vi "SDSU_DACS_ReadConstants.vi"(8 "error in (no error)":errorcluster, 11 "file path":path=path "/home/arcconfig/DHE_DACS.cfg") -> (0 "error out":errorcluster, 1 "number of dacs":i32, 2 "constants":string[][](table), 3 "resolutions":string[][](table), 4 "resolution":i32=4095)   [LabVIEW 2016]
uses:
  <vilib>/Utility/config.llb/Read Key (String).vi
  <vilib>/Utility/config.llb/Read Key (I32).vi
  <vilib>/Utility/config.llb/NI_LVConfig.lvlib
panel:
  # "off"
  # "curr"
  # "ll"
  # "type"
  # "def"
  # "ul"
  # "ll"
  # "b"
  # "comment"
  # "dn"
  # "gain"
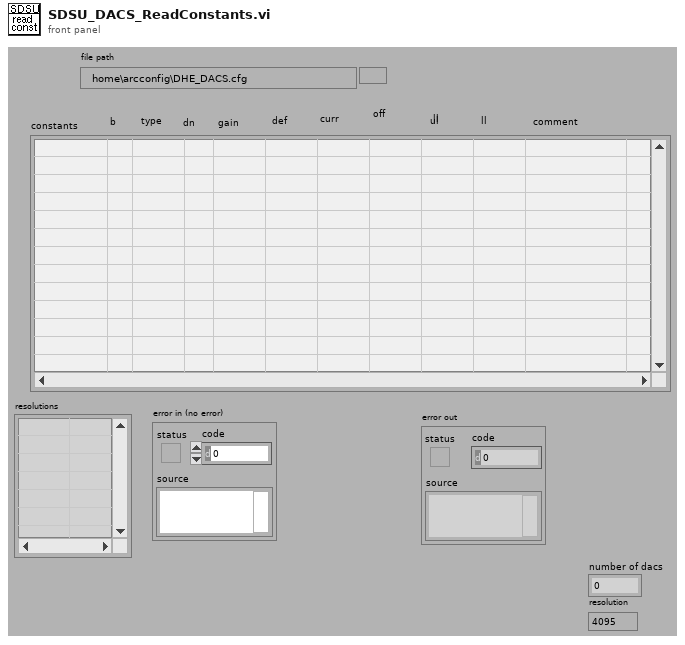
[diagram p1: front panel]
types:
  T1 = typedef "NI_LVConfig.lvlib/Config Data RefNum.ctl" = refnum<k1>
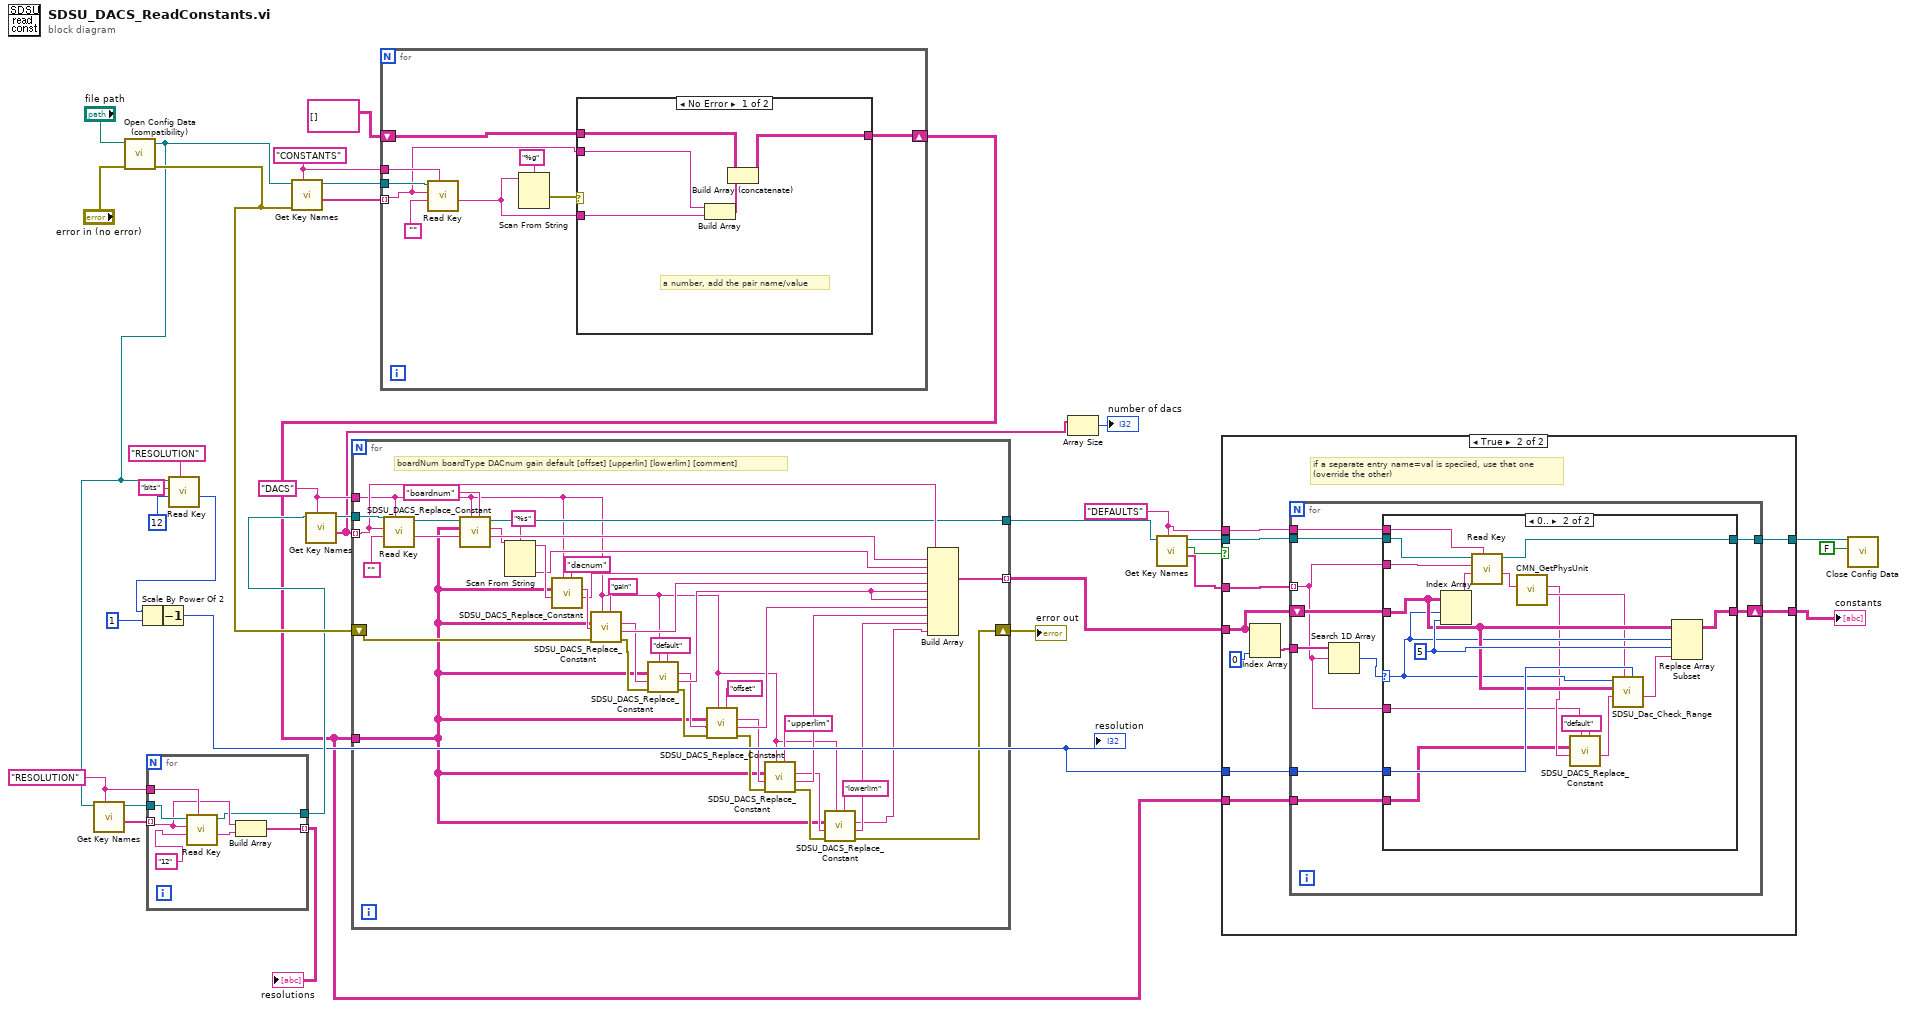
[diagram p0: block diagram]
diagram:
  w4 = "DEFAULTS" ("section")
  w14 = "RESOLUTION" ("section")
  w28 = "DACS" ("section")
  w35 = "CONSTANTS" ("section")
  n1 = call <vilib>:"Open Config Data (compatibility).vi"("error in (no error)"="error in (no error)", "configuration file path"="file path") -> ("error out"=w27:errorcluster, "refnum"=w16:T1)  [unwired: 7 in, 1 out]
  n2 = call <vilib>:"Get Key Names.vi"("section"=w14, "refnum"=w16) -> ("key names"=w15:string[], "refnum out"=w13:T1)  [unwired: 1 in, 7 out]
  n3 = for {
    tunnel: w15 -> [w38] mode=indexing
    tunnel: w14 -> [w42]
    tunnel: w13 -> [w40]
    tunnel: [w37] -> w11 mode=indexing
    tunnel: [w36] -> w12
    n4 = call-poly <vilib>:"Read Key.vi"("section"=w42, "default value"="12", "key"=w38, "refnum"=w40) -> ("value"=w39:string, "refnum out"=w36:T1)  [unwired: 2 in, 4 out]
    n5 = Build Array(w38, w39) -> (w37:string[])
  }
  "resolutions" <- w11
  n6 = call-poly <vilib>:"Read Key.vi"("section"="RESOLUTION", "default value"=12, "key"="bits", "refnum"=w16) -> ("value"=w20:i32)  [unwired: 1 in, 6 out]
  n7 = Scale By Power Of 2(n=w20, x=1) -> (x*2^n=w19:i32)
  n8 = Decrement(x=w19) -> (x-1=w2:i32)
  "resolution" <- w2
  n9 = call <vilib>:"Get Key Names.vi"("section"=w35, "error in (no error)"=w27, "refnum"=w16) -> ("key names"=w34:string[], "refnum out"=w31:T1)  [unwired: 7 out]
  n10 = call <vilib>:"Get Key Names.vi"("section"=w28, "refnum"=w12) -> ("key names"=w25:string[], "refnum out"=w29:T1)  [unwired: 1 in, 7 out]
  n11 = for {
    tunnel: w31 -> [w51]
    tunnel: w35 -> [w50]
    tunnel: w34 -> [w43] mode=indexing
    shift-right: [w48] -> w1
    shift-left: string[][] [] -> [w47]
    n12 = call-poly <vilib>:"Read Key.vi"("section"=w50, "default value"="", "key"=w43, "refnum"=w51) -> ("value"=w46:string)  [unwired: 2 in, 5 out]
    n13 = Scan From String(format string="%g", input string=w46) -> (error out=w44:errorcluster)  [unwired: 2 in, 4 out]
    n14 = case shown="No Error" w44 {
      tunnel: w43 -> [w56 _]
      tunnel: w46 -> [w55 _]
      tunnel: [w53 w57] -> w48
      tunnel: w47 -> [w52 w57]
      frame No Error {
        # "a number, add the pair name/value"
        n15 = Build Array(w56, w55) -> (w54:string[])
        n16 = Build Array (concatenate)(w52, w54) -> (w53:string[][])
      }
      frame Error {
        # "not a number\nskip it"
      }
    }
  }
  n17 = for {
    tunnel: w25 -> [w93] mode=indexing
    tunnel: w29 -> [w95]
    tunnel: w28 -> [w60]
    tunnel: [w88] -> w5 mode=indexing
    tunnel: w1 -> [w61]
    shift-right: [w75] -> w26
    shift-left: w27 -> [w91]
    tunnel: [w62] -> w10
    # "boardNum boardType DACnum gain default [offset] [upperlin] [lowerlim] [comment]"
    n18 = call-poly <vilib>:"Read Key.vi"("section"=w60, "default value"="", "key"=w93, "refnum"=w95) -> ("value"=w74:string, "refnum out"=w62:T1)  [unwired: 2 in, 4 out]
    n19 = call "SDSU_DACS_Replace_Constant.vi"("Field in"="boardnum", "DAC name"=w60, "value  in"=w74, "constants from file"=w61) -> ("value out"=w72:string, "rest out"=w71:string)  [unwired: 1 in, 5 out]
    n20 = Scan From String(format string="%s", input string=w71) -> (remaining string=w69:string, output 1=w68:string)  [unwired: 2 in, 3 out]
    n21 = call "SDSU_DACS_Replace_Constant.vi"("Field in"="dacnum", "DAC name"=w60, "value  in"=w69, "constants from file"=w61) -> ("value out"=w65:string, "rest out"=w66:string)  [unwired: 2 in, 4 out]
    n22 = call "SDSU_DACS_Replace_Constant.vi"("Field in"="gain", "DAC name"=w60, "error in (no error)"=w91, "value  in"=w66, "constants from file"=w61) -> ("error out"=w92:errorcluster, "value out"=w87:string, "rest out"=w64:string)  [unwired: 1 in, 3 out]
    n23 = call "SDSU_DACS_Replace_Constant.vi"("Field in"="default", "DAC name"=w60, "error in (no error)"=w92, "value  in"=w64, "constants from file"=w61) -> ("error out"=w76:errorcluster, "value out"=w86:string, "rest out"=w63:string)  [unwired: 1 in, 3 out]
    n24 = call "SDSU_DACS_Replace_Constant.vi"("Field in"="offset", "DAC name"=w60, "error in (no error)"=w76, "value  in"=w63, "constants from file"=w61) -> ("error out"=w90:errorcluster, "value out"=w85:string, "rest out"=w78:string)  [unwired: 1 in, 3 out]
    n25 = call "SDSU_DACS_Replace_Constant.vi"("Field in"="upperlim", "DAC name"=w60, "error in (no error)"=w90, "value  in"=w78, "constants from file"=w61) -> ("error out"=w89:errorcluster, "value out"=w84:string, "rest out"=w77:string)  [unwired: 1 in, 3 out]
    n26 = call "SDSU_DACS_Replace_Constant.vi"("Field in"="lowerlim", "DAC name"=w60, "error in (no error)"=w89, "value  in"=w77, "constants from file"=w61) -> ("error out"=w75:errorcluster, "value out"=w59:string, "rest out"=w58:string)  [unwired: 1 in, 3 out]
    n27 = Build Array(w93, w72, w68, w65, w87, w86, w86, w85, w84, w59, w58) -> (w88:string[])
  }
  "error out" <- w26
  n28 = Array Size(array=w25) -> (size(s)=→"number of dacs":i32)
  n29 = call <vilib>:"Get Key Names.vi"("section"=w4, "refnum"=w10) -> ("key names"=w6:string[], "section exists?"=w7:bool, "refnum out"=w9:T1)  [unwired: 1 in, 6 out]
  n30 = case shown="True" w7 {
    tunnel: w9 -> [w97 w104]
    tunnel: [w97 w101] -> w8
    tunnel: w6 -> [_ w107]
    tunnel: w5 -> [w96 w102]
    tunnel: w4 -> [_ w103]
    tunnel: [w96 w100] -> w3
    tunnel: w2 -> [_ w99]
    tunnel: w1 -> [_ w98]
    frame False {
    }
    frame True {
      # "if a separate entry name=val is speciied, use that one\n(override the other)"
      n31 = Index Array(array=w102, index (col)=0 ("index (row)")) -> (element=w105:string[])  [unwired: 1 in]
      n32 = for {
        tunnel: w107 -> [w109] mode=indexing
        tunnel: w105 -> [w117]
        tunnel: w104 -> [w115]
        tunnel: w103 -> [w114]
        shift-right: [w112] -> w100
        shift-left: w102 -> [w113]
        tunnel: [w111] -> w101
        tunnel: w99 -> [w110]
        tunnel: w98 -> [w108]
        n33 = Search 1D Array(1D array=w117, element=w109) -> (index of element=w116:i32)  [unwired: 1 out]
        n34 = case shown="0.." w116 {
          selector: w116 -> [_ w127]
          tunnel: w113 -> [w118 w128]
          tunnel: w115 -> [w119 w137]
          tunnel: w114 -> [_ w136]
          tunnel: w109 -> [_ w135]
          tunnel: [w118 w132] -> w112
          tunnel: [w119 w131] -> w111
          tunnel: w110 -> [_ w129]
          tunnel: w109 -> [_ w123]
          tunnel: w108 -> [_ w121]
          frame Default {
          }
          frame 0.. {
            w134 = 5 ("disabled index (col)")
            n35 = Index Array(array=w128, index (row)=w127, index (col)=w134) -> (element=w133:string)
            n36 = call-poly <vilib>:"Read Key.vi"("section"=w136, "default value"=w133, "key"=w135, "refnum"=w137) -> ("value"=w130:string, "refnum out"=w131:T1)  [unwired: 2 in, 4 out]
            n37 = call "CMN_GetPhysUnit.vi"("command in"=w130) -> ("unit"=w125:string, "command out"=w124:string)  [unwired: 9 out]
            n38 = call "SDSU_DACS_Replace_Constant.vi"("Field in"="default", "DAC name"=w123, "value  in"=w124, "constants from file"=w121) -> ("value out"=w120:string)  [unwired: 2 in, 5 out]
            n39 = call "SDSU_Dac_Check_Range.vi"("resolution"=w129, "unit"=w125, "value in"=w120, "DACS"=w128, "dac number"=w127) -> ("volts value"=w126:string)  [unwired: 1 in, 5 out]
            n40 = Replace Array Subset(array=w128, new element=w126, index (row)=w127, index (col)=w134) -> (w132:string[][])
          }
        }
      }
    }
  }
  "constants" <- w3
  n41 = call <vilib>:"Close Config Data.vi"("write file if changed (T)"=FALSE ("write configuration file? (T)"), "refnum"=w8) -> ()  [unwired: 1 in, 9 out]
